vi "Error Query.vi"(8 "error in (no error)":errorcluster, 11 "VISA resource name":refnum<visa-resource-name>) -> (0 "error out":errorcluster, 1 "Error Message":string, 2 "Error Code":i32[](array[numeric]), 3 "VISA resource name out":refnum<visa-resource-name>)   [LabVIEW 2018, in "Agilent MXA Series.lvlib"]
doc: "Queries the instrument for any errors in the instrument's error queue. It will continue to read errors until all errors have been read from the instrument. Any errors will be returned in the <B>error out</B> control.\n\n<B>Note:</B>\nThis VI is called automatically by most driver VIs so it is not usually necessary to call this in an application."
uses:
  Agilent MXA Series.lvlib
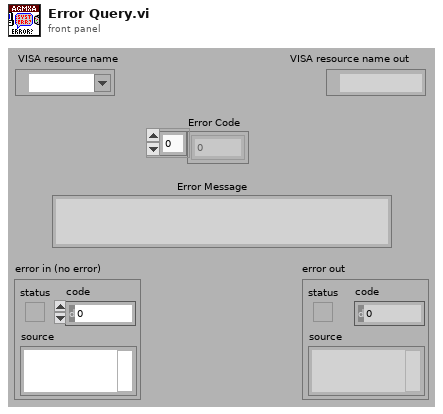
[diagram p1: front panel]
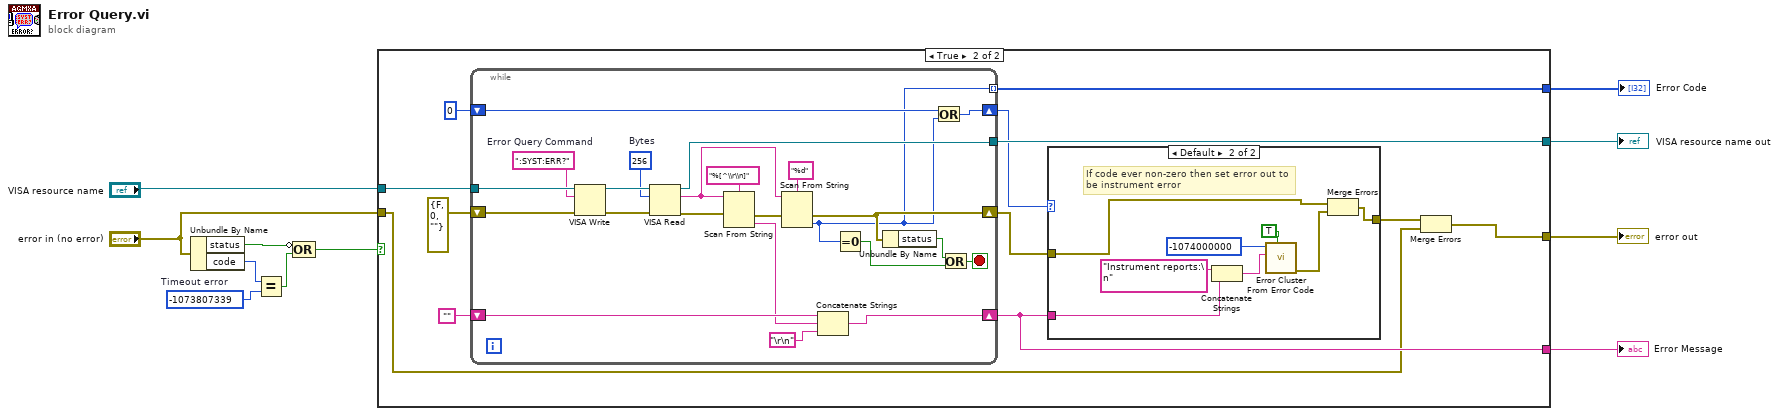
[diagram p0: block diagram]
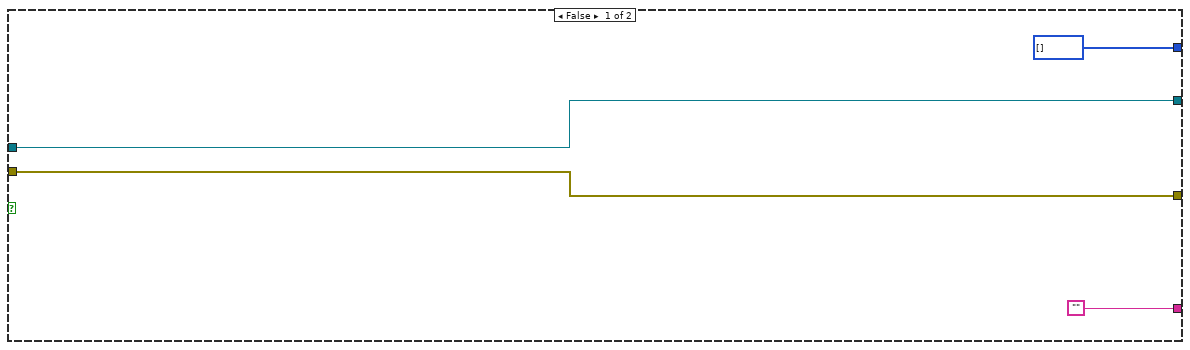
[diagram p2: hidden frame]
diagram:
  w10 = -1073807339  # Timeout error
  n1 = Unbundle By Name("error in (no error)") -> ("status"=w11:bool, "code"=w8:i32)
  n2 = Equal?(x=w8, y=w10) -> (x = y?=w9:bool)
  n3 = Compound Arithmetic op=OR(invert w11, w9) -> (w7:bool)
  n4 = case shown="True" w7 {
    tunnel: [w15 w27] -> w3
    tunnel: "VISA resource name" -> [w15 w26]
    tunnel: "error in (no error)" -> [w14 w18]
    tunnel: [w14 w24] -> w2
    tunnel: ["" w20] -> w1
    tunnel: [i32[] [] w19] -> w4
    frame False {
    }
    frame True {
      n5 = while {
        tunnel: [w59] -> w27
        tunnel: w26 -> [w58]
        shift-right: [w46] -> w20
        shift-left: "" -> [w49]
        shift-right: [w40] -> w16
        shift-left: i16 0 -> [w39]
        shift-right: [w44] -> w17
        shift-left: errorcluster {"status"=FALSE, "code"=0, "source"=""} ("error in (no error)") -> [w45]
        tunnel: [w37] -> w19 mode=indexing
        stop <- w52 stop-if-true
        w56 = u32 256  # Bytes
        w54 = ":SYST:ERR?"  # Error Query Command
        n6 = VISA Write(VISA resource name=w58, write buffer=w54, error in (no error)=w45) -> (VISA resource name out=w57:refnum<visa-resource-name>, error out=w55:errorcluster)  [unwired: 1 out]
        n7 = VISA Read(VISA resource name=w57, byte count=w56, error in (no error)=w55) -> (VISA resource name out=w59:refnum<visa-resource-name>, read buffer=w50:string, error out=w43:errorcluster)  [unwired: 1 out]
        n8 = Scan From String(format string="%[^\\r\\n]", input string=w50, error in=w43) -> (error out=w42:errorcluster, output 1=w47:string)  [unwired: 2 in, 2 out]
        n9 = Scan From String(format string="%d", input string=w50, error in=w42) -> (error out=w44:errorcluster, output 1=w37:i32)  [unwired: 2 in, 2 out]
        n10 = Concatenate Strings(w49, w47, "\r\n") -> (w46:string)
        n11 = Equal To 0?(x=w37) -> (x = 0?=w38:bool)
        n12 = Unbundle By Name(w44) -> ("status"=w41:bool)
        n13 = Or(x=w39, y=w37) -> (x .or. y?=w40:i32)
        n14 = Or(x=w41, y=w38) -> (x .or. y?=w52:bool)
      }
      n15 = case shown="Default" w16 {
        tunnel: w20 -> [_ w35]
        tunnel: [w28 w29] -> w22
        tunnel: w17 -> [w28 w30]
        frame 0 {
        }
        frame Default {
          # "If code ever non-zero then set error out to\nbe instrument error"
          n16 = Concatenate Strings("Instrument reports:\n" ("Source"), w35) -> (w33:string)
          n17 = call <vilib>:"Error Cluster From Error Code.vi"("show call chain? (False)"=TRUE, "error message (\"\")"=w33, "error code (0)"=-1074000000 ("Code")) -> ("error out"=w31:errorcluster)  [unwired: 6 in]
          n18 = Merge Errors(w30, w31) -> (w29:errorcluster)
        }
      }
      n19 = Merge Errors(w22, w18) -> (w24:errorcluster)
    }
  }
  "VISA resource name out" <- w3
  "error out" <- w2
  "Error Message" <- w1
  "Error Code" <- w4
